vi "Get View VI Reference.vi"(8 "error in (no error)":errorcluster, 11 "View In":refnum<class "View.lvclass">) -> (0 "error out":errorcluster, 2 "View VI Reference":refnum<vi>, 3 "View Out":refnum<class "View.lvclass">)   [LabVIEW 2020, in "View.lvclass"]
doc: "Get the View VI referene as set by the Set View VI Reference.vi method."
uses:
  View.lvclass
  C:/git/astemes-triarc-framework/source/Framework/Process/Process.lvclass
  Process/Process.lvclass/Process.ctl
  View.lvclass/View.ctl
  Process/Protected/Messaging/Async Request Message.vi
  Process/Private/SubVIs/Handle Debug Data.vi
  Logging/Log Debug.vi
  <vilib>/AdvancedString/1D String Array to Delimited String.vi
  <vilib>/Utility/High Resolution Relative Seconds.vi
  Synchronous Request Callback/Synchronous Request Callback.lvclass
  C:/git/astemes-triarc-framework/source/Framework/Callback/Callback.lvclass
  Process/Process.lvclass
  C:/git/astemes-triarc-framework/source/Framework/Logging/Logging.lvclass
  <vilib>/Utility/error.llb/Error Cluster From Error Code.vi
  Synchronous Request Callback/Create.vi
  Process/Public/Read Name.vi
  Process/Private/SubVIs/Wait for Response Message.vi
  Callback/Callback.lvclass
  Logging/Logging.lvclass
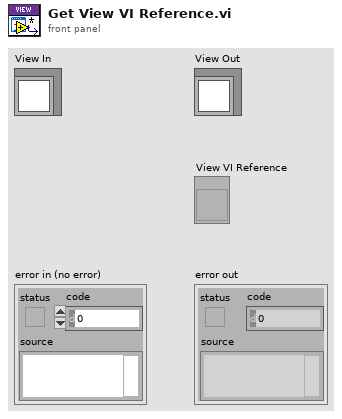
[diagram p1: front panel]
types:
  T1 = typedef "Process.lvclass/API Mode.ctl" = enum16{"Send Message", "Handle Message"}
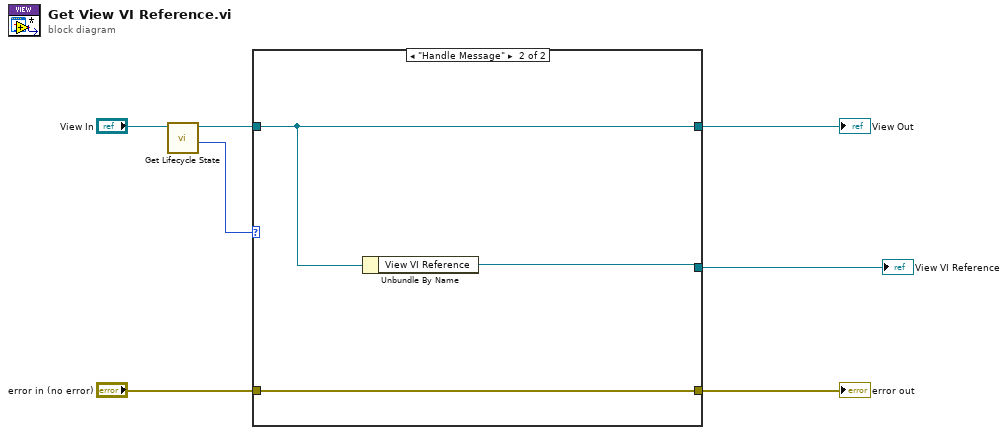
[diagram p0: block diagram]
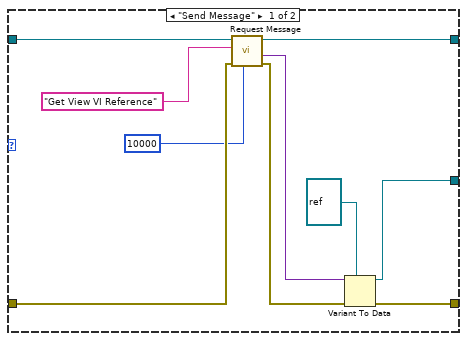
[diagram p2: hidden frame]
diagram:
  n1 = call "Get Lifecycle State.vi"("Process In"="View In") -> ("API Mode"=w2:T1, "Process Out"=w3:refnum<class "View.lvclass">)  [unwired: 7 in, 2 out]
  n2 = case shown="\"Handle Message\"" w2 {
    tunnel: [w17 w19] -> w6
    tunnel: [w14 w18] -> w5
    tunnel: [w11 w20] -> w4
    tunnel: w3 -> [w10 w19]
    tunnel: "error in (no error)" -> [w9 w18]
    frame "Send Message" {
      n3 = call "Request Message.vi"("timeout in ms (-1)"=10000, "error in (no error)"=w9, "Request Message"="Get View VI Reference", "Process In"=w10) -> ("error out"=w16:errorcluster, "Response Message Data"=w12:variant, "Process Out"=w17:refnum<class "View.lvclass">)  [unwired: 3 in, 2 out]
      n4 = Variant To Data(error in=w16, type=refnum<vi> refnum ("UI View VI Reference"), Variant=w12) -> (data=w11:refnum<vi>, error out=w14:errorcluster)
    }
    frame "Handle Message" {
      n5 = Unbundle By Name(w19) -> ("View VI Reference"=w20:refnum<vi>)
    }
  }
  "error out" <- w5
  "View Out" <- w6
  "View VI Reference" <- w4
